vi "CC Script Parse Telescope Focus Move.vi"(8 "error in (no error)":errorcluster, 9 "To Script?":bool, 10 "Telescope Move Pos":dbl, 11 "Telescope Move Parameters":string="Motor=2") -> (0 "error out":errorcluster, 2 "Script Out":string="ObjectName \"RA\":\"123.456\",\"DEC\":\"4546.54\"", 3 "Telescope Move Pos":dbl)   [LabVIEW 2021]
uses:
  <vilib>/regexp/Match Regular Expression.xnode
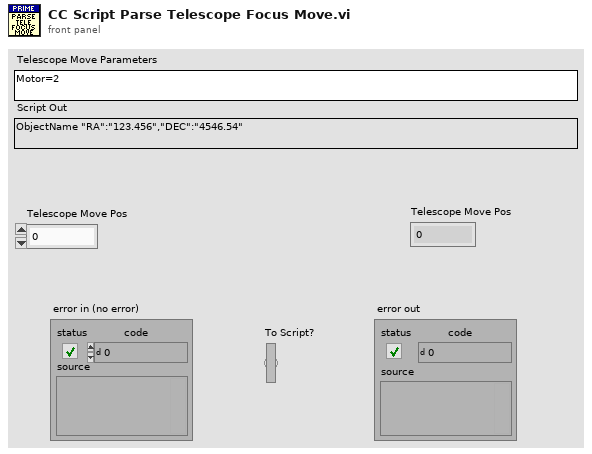
[diagram p1: front panel]
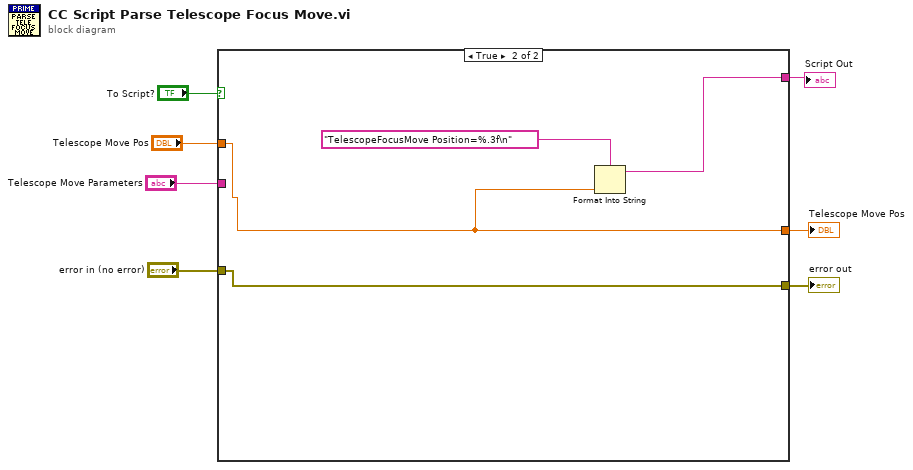
[diagram p0: block diagram]
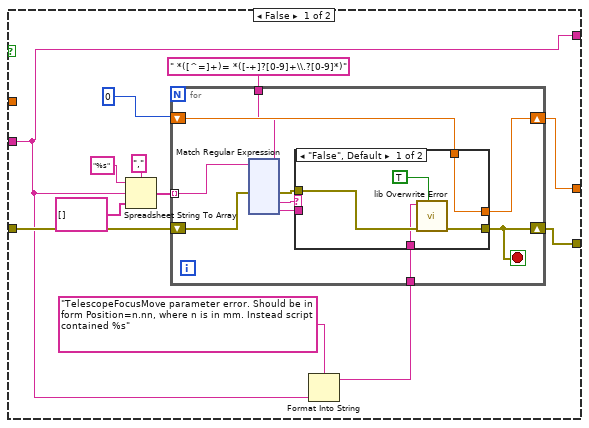
[diagram p2: hidden frame]
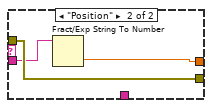
[diagram p3: hidden frame]
diagram:
  n1 = case shown="True" "To Script?" {
    tunnel: [w19 w158] -> w7
    tunnel: "error in (no error)" -> [w18 w159]
    tunnel: [w10 w159] -> w5
    tunnel: "Telescope Move Parameters" -> [w13 _]
    tunnel: "Telescope Move Pos" -> [_ w158]
    tunnel: [w13 w160] -> w2
    frame False {
      n2 = Spreadsheet String To Array(delimiter (Tab)=",", format string="%s", spreadsheet string=w13, array type (2D Dbl)=string[] []) -> (array=w12:string[])
      n3 = Format Into String(format string="TelescopeFocusMove parameter error. Should be in form Position=n.nn, where n is in mm. Instead script contained %s", w13) -> (resulting string=w11:string)  [unwired: 2 in, 1 out]
      n4 = for {
        shift-right: [w28] -> w19
        shift-left: 0 -> [w29]
        tunnel: w12 -> [w27] mode=indexing
        tunnel: w11 -> [w22]
        shift-right: [w21] -> w10
        shift-left: w18 -> [w24]
        tunnel: " *([^=]+)= *([-+]?[0-9]+\\.?[0-9]*)" ("format string") -> [w20]
        stop <- w21 stop-if-true
        n5 = xnode "Match Regular Expression"("input string"=w27, "regular expression"=w20, "error in"=w24) -> ("error out"=w23:errorcluster, "submatch 1"=w26:string, "submatch 2"=w25:string)  [unwired: 3 in, 4 out]
        n6 = case shown="\"False\", Default" w26 {
          tunnel: w29 -> [w31 _]
          tunnel: [w31 w35] -> w28
          tunnel: w25 -> [_ w36]
          tunnel: w23 -> [w34 w37]
          tunnel: w22 -> [w33 _]
          tunnel: [w32 w37] -> w21
          frame "False", Default {
            n7 = call "lib Overwrite Error.vi"("Force Error?"=TRUE, "error in (no error)"=w34, "Error Message"=w33) -> ("error out"=w32:errorcluster)  [unwired: 8 in]
          }
          frame "Position" {
            n8 = Fract/Exp String To Number(string=w36) -> (number=w35:dbl)  [unwired: 3 in, 1 out]
          }
        }
      }
    }
    frame True {
      n9 = Format Into String(format string="TelescopeFocusMove Position=%.3f\n", w158) -> (resulting string=w160:string)  [unwired: 2 in, 1 out]
    }
  }
  "error out" <- w5
  "Telescope Move Pos" <- w7
  "Script Out" <- w2
